vi "08_dosing.vi"() -> ()   [LabVIEW 2024]
uses:
  <vilib>/Utility/error.llb/DialogType.ctl
  0fc544a7-5f76-4a6f-b25e-3c23831dfa25.vi
  4067e6f5-c9bb-441e-8d38-abed3cce061a.vi
  <vilib>/Waveform/WDTOps.llb/WDT Waveform to XY Pairs DBL.vi
  <instrlib>/Tektronix DMM40x0 Series/Tektronix DMM40x0 Series.lvlib
panel:
  out "Waveform Graph 2":dbl[](array[numeric])
  out "STABLE":bool
  in  "Serial Communication":T1={"Baud Rate"=9600, "Parity"=0, "Data Bits"=8, "Stop Bits"=10, "Flow Control"=0} {"Flow Control" items=["None", "XON/XOFF", "RTS/CTS", "XON/XOFF & RTS/CTS", "DTR/DSR", "XON/XOFF & DTR/DSR"]; "Stop Bits" items=["1.0"=10, "1.5"=15, "2.0"=20]; "Data Bits" items=["7"=7, "8"=8]; "Parity" items=["None", "Odd", "Even", "Mark", "Space"]; "Baud Rate" items=["300"=300, "600"=600, "1200"=1200, "2400"=2400, "4800"=4800, "9600"=9600, "19200"=19200]}
  in  "COM PORT (COM2)":refnum<visa-resource-name>
  out "Stability threshold":dbl format="%#_13g"
  out "Waveform Graph":dbl[](graph)
  # "Voltmeter Serial Configuration"
  # "DEFAULT SETTINGS:\n\nTimeout (10000 ms)\nTrigger Count (5000)\nSample Count (1)\n\n****DC VOLTAGE***"
  # "Voltmeter Stability"
  # "0 - Stability threshold not met\n1 - Stability threshold met\n\n\n\n*stability (+/-0.05 mV) of last 15 pts"
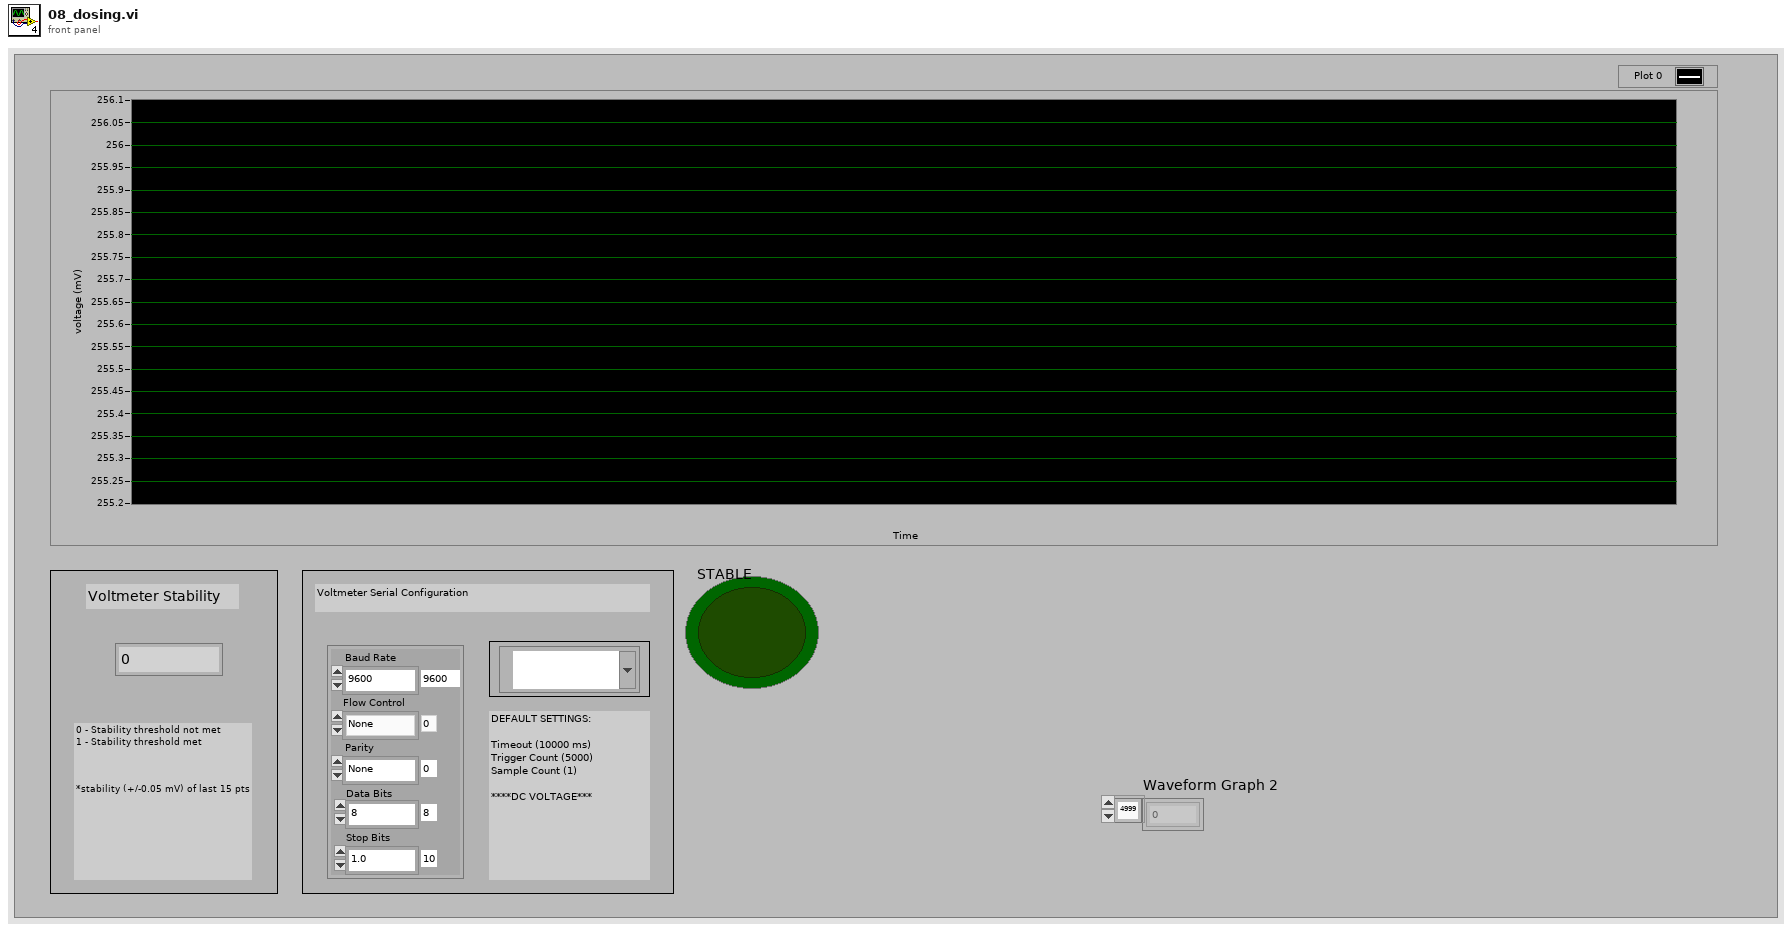
[diagram p1: front panel]
types:
  T1 = cluster{"Baud Rate":u32, "Parity":u16, "Data Bits":u16, "Stop Bits":u16, "Flow Control":u16}
  T2 = typedef "DialogType.ctl" = u16
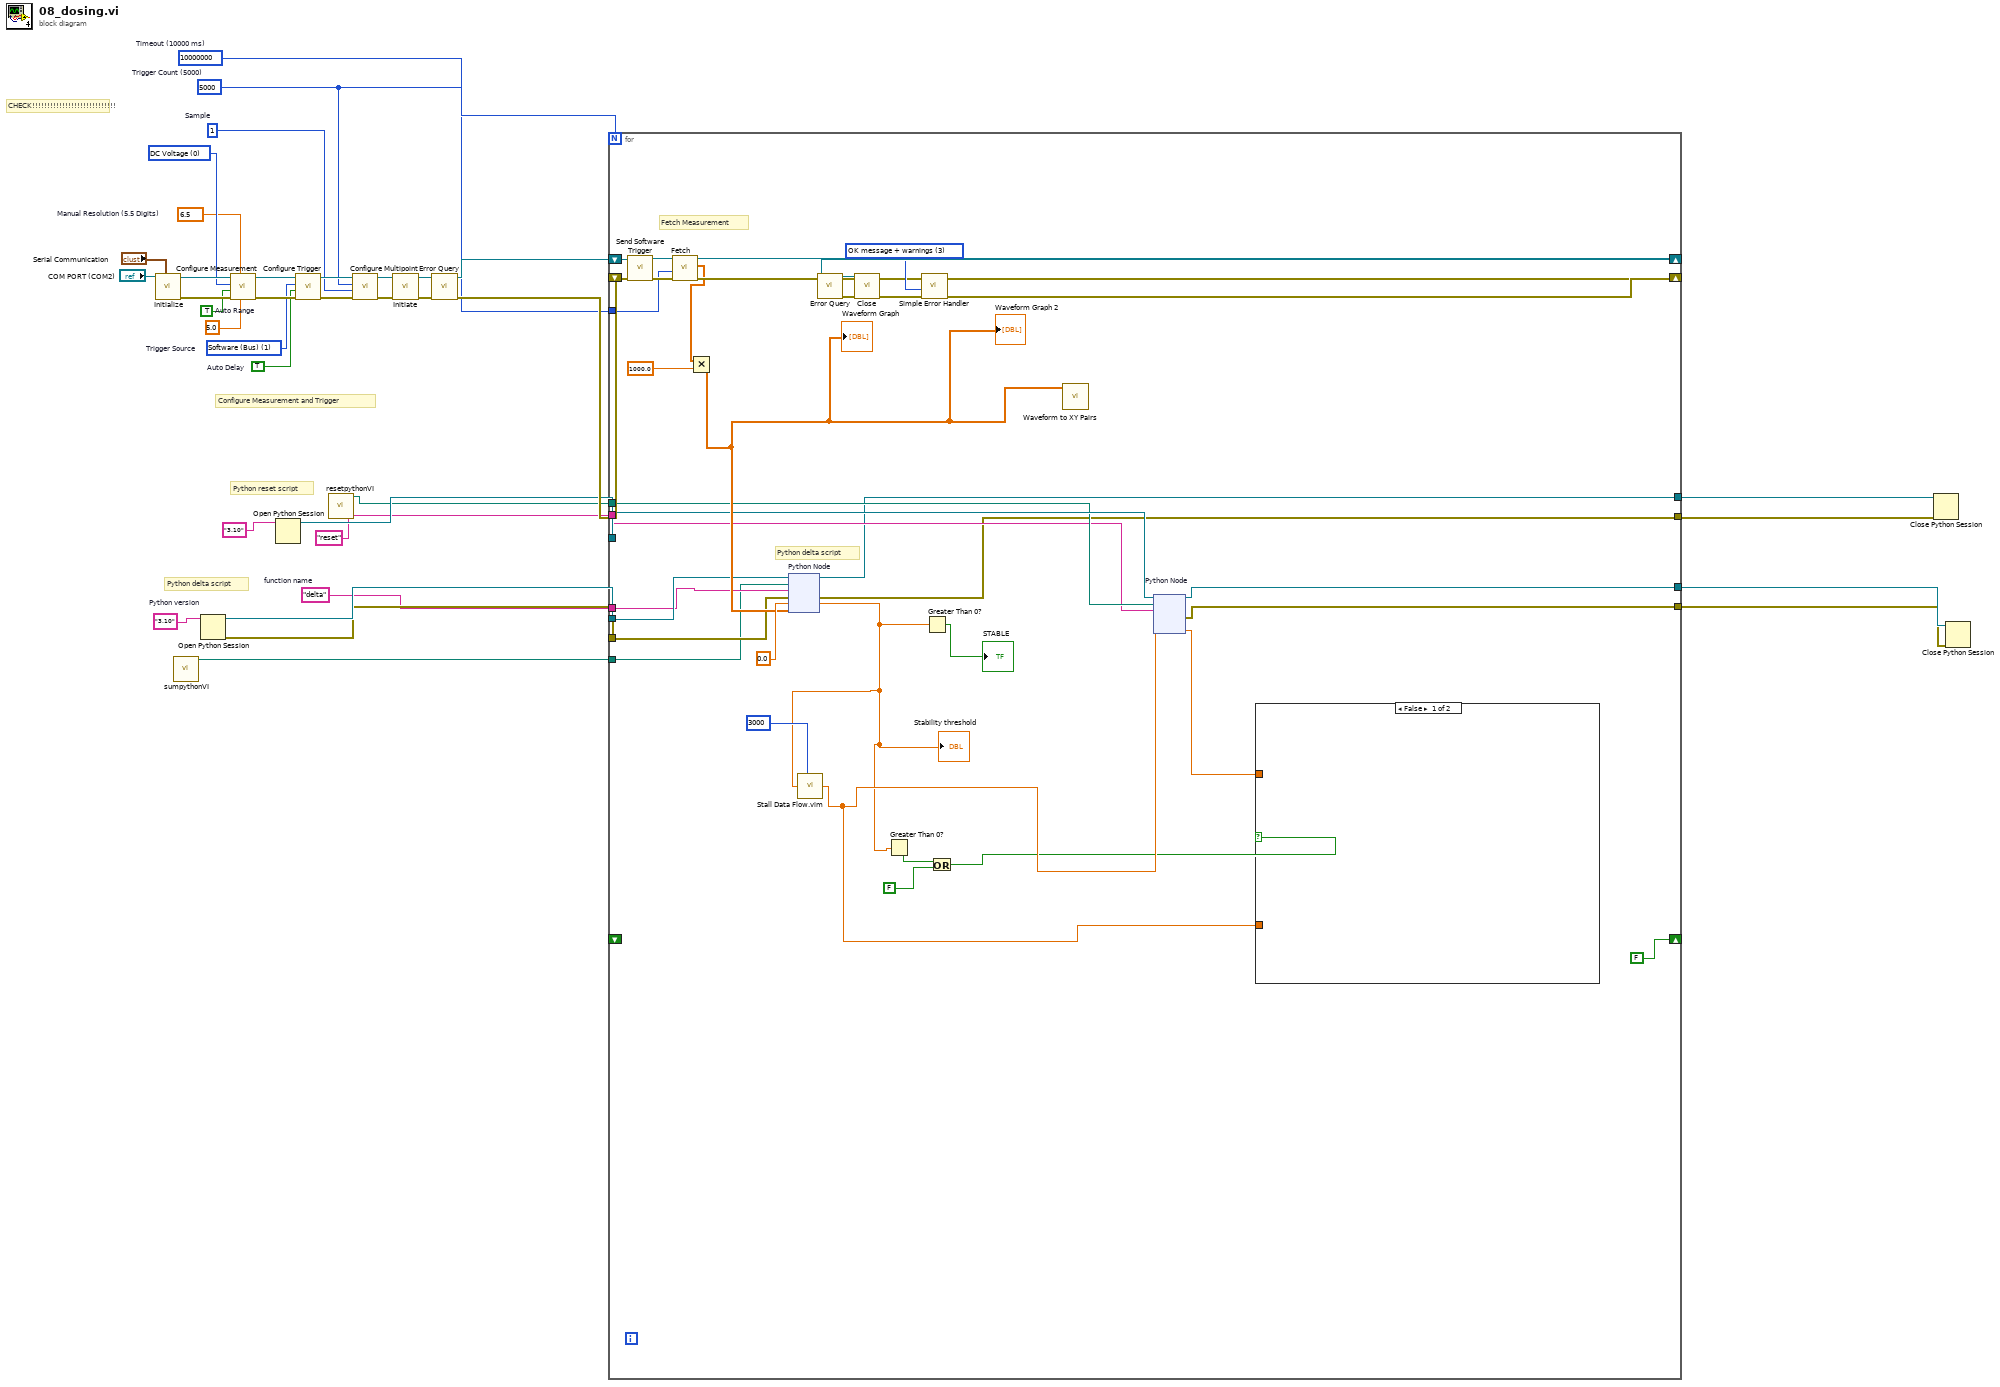
[diagram p0: block diagram]
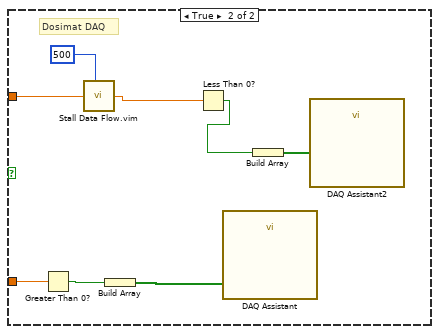
[diagram p2: hidden frame]
diagram:
  w1 = T2 3 items=["no dialog", "OK message", "continue or stop message", "OK message + warnings", "continue/stop + warnings"] ("type of dialog (OK msg:1)")
  w14 = "delta"  # function name
  w17 = "3.10"  # Python version
  w29 = u16 0 items=["DC Voltage", "AC Voltage", "2 - Wire Resistance", "4 - Wire Resistance", "DC Current", "AC Current", "Frequency", "Period", "Continuity", "Diode Checking", "Temperature", "Capacitance"] ("Function (0: DC Voltage)")
  w20 = u32 10000000  # Timeout (10000 ms)
  w21 = 1  # Sample
  w28 = 5000  # Trigger Count (5000)
  w22 = 6.5 items=["4.5"=4.5, "5.5"=5.5, "6.5"=6.5]  # Manual Resolution (5.5 Digits)
  w30 = TRUE  # Auto Delay
  w31 = u16 1 items=["Immediate", "Software (Bus)", "External"]  # Trigger Source
  w32 = TRUE  # Auto Range
  # "Python delta script"
  # "Python reset script"
  # "CHECK!!!!!!!!!!!!!!!!!!!!!!!!!!!!"
  # "Configure Measurement and Trigger"
  n1 = call <instrlib>:"Initialize.vi"("Serial Configuration"="Serial Communication", "VISA resource name"="COM PORT (COM2)") -> ("error out"=w41:errorcluster, "VISA resource name out"=w42:refnum<visa-resource-name>)  [unwired: 3 in, 5 out]
  n2 = call "sumpythonVI.vi"() -> ("appended path"=w13:path)  [unwired: 11 in]
  n3 = Open Python Session(python version=w17) -> (session out=w19:refnum<k35>, error out=w18:errorcluster)  [unwired: 2 in]
  n4 = call <instrlib>:"Configure Measurement.vi"("Manual Range (1.0)"=5.0, "Manual Resolution (5.5 Digits)"=w22, "error in (no error)"=w41, "Auto Range (T:Enable)"=w32, "Function (0: DC Voltage)"=w29, "VISA resource name"=w42) -> ("error out"=w39:errorcluster, "VISA resource name out"=w40:refnum<visa-resource-name>)  [unwired: 4 out]
  n5 = Open Python Session(python version="3.10" ("Python version")) -> (session out=w15:refnum<k35>)  [unwired: 2 in, 1 out]
  n6 = call <instrlib>:"Configure Trigger.vi"("error in (no error)"=w39, "Auto Delay (T: Enable)"=w30, "Trigger Source (0: Immediate)"=w31, "VISA resource name"=w40) -> ("error out"=w37:errorcluster, "VISA resource name out"=w38:refnum<visa-resource-name>)  [unwired: 1 in, 5 out]
  n7 = call "resetpythonVI.vi"() -> ("appended path"=w12:path)  [unwired: 11 in]
  n8 = call <instrlib>:"Configure Multipoint.vi"("error in (no error)"=w37, "Sample Count (1)"=w21, "Trigger Count (1)"=w28, "VISA resource name"=w38) -> ("error out"=w35:errorcluster, "VISA resource name out"=w36:refnum<visa-resource-name>)  [unwired: 6 out]
  n9 = call <instrlib>:"Initiate.vi"("error in (no error)"=w35, "VISA resource name"=w36) -> ("error out"=w27:errorcluster, "VISA resource name out"=w26:refnum<visa-resource-name>)  [unwired: 8 out]
  n10 = call <instrlib>:"Error Query.vi"("error in (no error)"=w27, "VISA resource name"=w26) -> ("error out"=w24:errorcluster, "VISA resource name out"=w25:refnum<visa-resource-name>)  [unwired: 8 out]
  n11 = for {
    N: w28 -> [_]
    shift-right: [w72] -> w3
    shift-left: w24 -> [w68]
    shift-right: [w73] -> w5
    shift-left: w25 -> [w69]
    tunnel: w20 -> [w67]
    tunnel: w19 -> [w60]
    tunnel: w18 -> [w59]
    tunnel: w15 -> [w58]
    tunnel: w14 -> [w57]
    tunnel: w13 -> [w56]
    tunnel: w12 -> [w55]
    tunnel: "reset" ("function name") -> [w54]
    tunnel: [w53] -> w10
    tunnel: [w52] -> w9
    tunnel: [w51] -> w8
    tunnel: [w50] -> w7
    shift-right: [FALSE] -> _
    shift-left: _ -> [_]
    # "Python delta script"
    # "Fetch Measurement"
    n12 = call <instrlib>:"Send Software Trigger.vi"("error in (no error)"=w68, "VISA resource name"=w69) -> ("error out"=w70:errorcluster, "VISA resource name out"=w71:refnum<visa-resource-name>)  [unwired: 8 out]
    n13 = call <instrlib>:"Fetch.vi"("error in (no error)"=w70, "Timeout (10000 ms)"=w67, "VISA resource name"=w71) -> ("error out"=w72:errorcluster, "Measurements"=w65:dbl[], "VISA resource name out"=w73:refnum<visa-resource-name>)  [unwired: 6 out]
    n14 = Multiply(x=w65, y=1000.0) -> (x*y=w64:dbl[])
    "Waveform Graph" <- w64
    "Waveform Graph 2" <- w64
    n15 = node "Python Node"(w60, w56, w57, w59, 0.0, w64) -> (w51:refnum<k35>, w50:errorcluster, w45:dbl)  [unwired: 1 in, 2 out]
    "Stability threshold" <- w45
    n16 = call "Stall Data Flow.vim"("value in"=w45, "milliseconds to wait"=u32 3000) -> ("value out"=w47:dbl)  [unwired: 1 out]
    n17 = Greater Than 0?(x=w45) -> (x > 0?=w44:bool)
    n18 = Greater Than 0?(x=w45) -> (x > 0?=→"STABLE":bool)
    n19 = Or(x=w44, y=FALSE) -> (x .or. y?=w43:bool)
    n20 = call-poly <vilib>:"Waveform to XY Pairs.vi"("waveform in"=w64) -> ()  [unwired: 8 in, 3 out]
    n21 = node "Python Node"(w58, w55, w54, w47) -> (w53:refnum<k35>, w52:errorcluster, w61:dbl)  [unwired: 3 in, 2 out]
    n22 = case shown="False" w43 {
      tunnel: w47 -> [_ w79]
      tunnel: w61 -> [_ w75]
      frame False {
      }
      frame True {
        # "Dosimat DAQ"
        n23 = Greater Than 0?(x=w79) -> (x > 0?=w78:bool)
        n24 = call "Stall Data Flow.vim"("value in"=w75, "milliseconds to wait"=u32 500) -> ("value out"=w76:dbl)  [unwired: 1 out]
        n25 = Build Array(w78) -> (w77:bool[])
        n26 = Less Than 0?(x=w76) -> (x < 0?=w80:bool)
        n27 = call "DAQ Assistant"("data"=w77) -> ()  [unwired: 17 in, 2 out]
        n28 = Build Array(w80) -> (w81:bool[])
        n29 = call "DAQ Assistant2"("data"=w81) -> ()  [unwired: 17 in, 2 out]
      }
    }
  }
  n30 = call <instrlib>:"Error Query.vi"("error in (no error)"=w3, "VISA resource name"=w5) -> ("error out"=w2:errorcluster, "VISA resource name out"=w4:refnum<visa-resource-name>)  [unwired: 8 out]
  n31 = call <instrlib>:"Close.vi"("error in (no error)"=w2, "VISA resource name"=w4) -> ("error out"=w6:errorcluster)  [unwired: 9 out]
  n32 = call <vilib>:"Simple Error Handler.vi"("type of dialog (OK msg:1)"=w1, "error in (no error)"=w6) -> ()  [unwired: 8 out]
  n33 = Close Python Session(session in=w8, error in=w7) -> ()  [unwired: 1 out]
  n34 = Close Python Session(session in=w10, error in=w9) -> ()  [unwired: 1 out]
